vi "h.ACQ.ParseGetPeaksHeader.vi"(11 "Header from #GetPeaks":u8[](array[numeric])) -> (0 "Header Version":u16, 1 "Time Stamp (ns)":u64, 2 "SN":u64, 3 "Header Length":u16, 4 "#Peaks":u16[](array[numeric]))   [LabVIEW 2019, in "h.Library.lvlib"]
doc: "This vi parses the header returned by the #GetPeaks command and returns the contained data through a number of outputs.\n\n<b>Header from #GetPeaks</b> - data returned by #GetPeaks.vi\n<b>Header Version</b> - Version number of the header\n<b>Header Length</b> - The total header length in bytes (also the start of the peaks data)s\n<b>SN</b> - Serial Number of the collected data set\n<b>Time Stamp</b> - The estimated time in ns when the instrument acquired the spectrum\n<b>#Peaks</b> - Array containing the number of detected peaks on each channel"
uses:
  h.Library.lvlib
panel:
  out "Reserved":u32
  # "Hyperion Parse #GetPeaks Header"
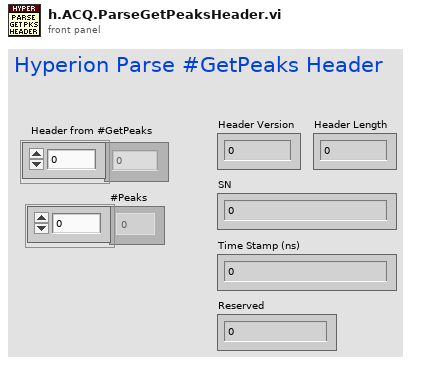
[diagram p1: front panel]
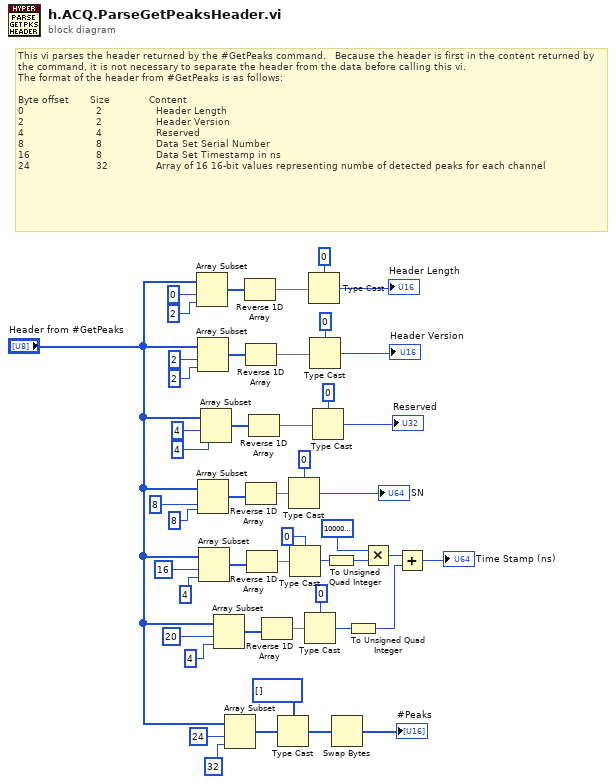
[diagram p0: block diagram]
diagram:
  # "This vi parses the header returned by the #GetPeaks command.   Because the header is first in the content returned by the command, it is not necessary to separate the header from the data before calling this vi.\nThe format of the header from #GetPeaks is as follows:\n\nByte offset       Size             Content\n0                        2                  Header Length\n2                        2                  Header Version\n4                        4                  Reserved\n8                        8                  Data Set Serial Number\n16                      8                  Data Set Timestamp in ns\n24                      32                Array of 16 16-bit values representing numbe of detected peaks for each channel"
  n1 = Array Subset(array="Header from #GetPeaks", index=0, length=2) -> (w12:u8[])
  n2 = Array Subset(array="Header from #GetPeaks", index=2, length=2) -> (w38:u8[])
  n3 = Array Subset(array="Header from #GetPeaks", index=8, length=8) -> (w25:u8[])
  n4 = Array Subset(array="Header from #GetPeaks", index=16, length=4) -> (w19:u8[])
  n5 = Array Subset(array="Header from #GetPeaks", index=4, length=4) -> (w4:u8[])
  n6 = Array Subset(array="Header from #GetPeaks", index=20, length=4) -> (w41:u8[])
  n7 = Array Subset(array="Header from #GetPeaks", index=24, length=32 ("y")) -> (w9:u8[])
  n8 = Reverse 1D Array(array=w12) -> (reversed array=w13:u8[])
  n9 = Reverse 1D Array(array=w38) -> (reversed array=w39:u8[])
  n10 = Reverse 1D Array(array=w25) -> (reversed array=w24:u8[])
  n11 = Reverse 1D Array(array=w19) -> (reversed array=w21:u8[])
  n12 = Reverse 1D Array(array=w4) -> (reversed array=w5:u8[])
  n13 = Reverse 1D Array(array=w41) -> (reversed array=w31:u8[])
  n14 = Type Cast(type=u16[] [], x=w9) -> (*(type *) &x=w44:u16[])
  n15 = Type Cast(type=u64 0 ("length"), x=w24) -> (*(type *) &x=→"SN":u64)
  n16 = Type Cast(type=u32 0 ("length"), x=w21) -> (*(type *) &x=w36:u32)
  n17 = Type Cast(type=u32 0 ("length"), x=w31) -> (*(type *) &x=w35:u32)
  n18 = Type Cast(type=u16 0 ("length"), x=w13) -> (*(type *) &x=→"Header Length":u16)
  n19 = Type Cast(type=u16 0 ("length"), x=w39) -> (*(type *) &x=→"Header Version":u16)
  n20 = Type Cast(type=u32 0 ("length"), x=w5) -> (*(type *) &x=→"Reserved":u32)
  n21 = To Unsigned Quad Integer(1:w36) -> (0:w47:u64)
  n22 = Swap Bytes(anything=w44) -> (byte swapped=→"#Peaks":u16[])
  n23 = To Unsigned Quad Integer(1:w35) -> (0:w34:u64)
  n24 = Multiply(x=u64 1000000000 ("y"), y=w47) -> (x*y=w33:u64)
  n25 = Add(x=w33, y=w34) -> (x+y=→"Time Stamp (ns)":u64)
